vi "RGBC_init.vi"(11 "Channel Name":tag="B/I2C") -> (0 "error out":errorcluster, 3 "I2C Ref Out":T1={"myRIO Reference"={"myRIO Model"=enum."Unknown", "myRIO Hardware Reference"={"Generic FPGA Reference"=refnum, "Allow multiple opens"=FALSE}}, "I2C Channels Enum"=enum."Not Connected", "I2C Configuration"={"I2C Transfer Rate"=enum."Fast mode (400 kbps)"}})   [LabVIEW 2017]
uses:
  <vilib>/myRIO/Instrument Drivers/Onboard IO/I2C/typedefs/I2C Reference.ctl
  <vilib>/myRIO/Common/Instrument Driver Framework/Utilities/typedefs/myRIO Generic Hardware Reference.ctl
  <vilib>/myRIO/Common/Instrument Driver Framework/Utilities/typedefs/Hardware Version Enum.ctl
  <vilib>/myRIO/Common/Instrument Driver Framework/Utilities/typedefs/myRIO v1.0 Reference.ctl
  <vilib>/myRIO/Common/Instrument Driver Framework/Utilities/typedefs/Generic FPGA Reference.ctl
  <vilib>/myRIO/Common/Instrument Driver Framework/myRIO v1.0/I2C/typedefs/I2C Channels Enum.ctl
  <vilib>/myRIO/Instrument Drivers/Onboard IO/I2C/typedefs/I2C Configuration.ctl
  <vilib>/myRIO/Instrument Drivers/Onboard IO/I2C/typedefs/I2C Transfer Rate.ctl
  <vilib>/myRIO/Instrument Drivers/Onboard IO/I2C/typedefs/I2C User Configuration.ctl
  <vilib>/Utility/error.llb/Error Cluster From Error Code.vi
  <vilib>/myRIO/Common/Instrument Driver Framework/myRIO v1.0/I2C/vis/myRIO v1.0 Configure I2C.vi
  <vilib>/myRIO/Common/Instrument Driver Framework/myRIO v1.0/I2C/vis/myRIO v1.0 Write I2C.vi
  <vilib>/myRIO/Common/Instrument Driver Framework/myRIO v1.0/I2C/vis/myRIO v1.0 Read I2C.vi
  <vilib>/myRIO/Instrument Drivers/Onboard IO/I2C/I2C.lvlib
panel:
  in  "error in (no error)":errorcluster
  # "2981 EB8F 0180 0180 83"
  # "Set gain"
  # "Gain"
  # "Set enable"
  # "Enable"
  # "Set enable"
  # "Enable/timer on"
  # "Set integration time"
  # "Integration Time"
  # "Check for sensor"
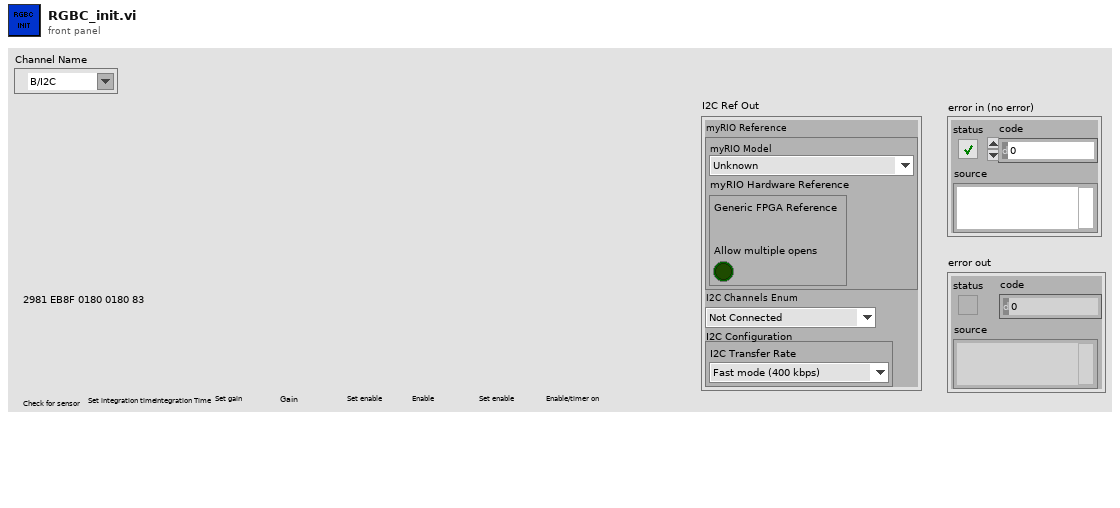
[diagram p1: front panel]
types:
  T1 = typedef "I2C.lvlib/I2C Reference.ctl" = cluster{"myRIO Reference":T2, "I2C Channels Enum":T6, "I2C Configuration":T7}
  T2 = typedef "myRIO Generic Hardware Reference.ctl" = cluster{"myRIO Model":T3, "myRIO Hardware Reference":T4}
  T3 = typedef "Hardware Version Enum.ctl" = enum16{"Unknown", "myRIO-1900", "myRIO-1950", "roboRIO", "NI ELVIS RIO CM"}
  T4 = typedef "myRIO v1.0 Reference.ctl" = cluster{"Generic FPGA Reference":T5, "Allow multiple opens":bool}
  T5 = typedef "Generic FPGA Reference.ctl" = refnum<k20>
  T6 = typedef "I2C Channels Enum.ctl" = enum16{"Not Connected", "A/I2C", "B/I2C", "I2C/I2C"}
  T7 = typedef "I2C.lvlib/I2C Configuration.ctl" = cluster{"I2C Transfer Rate":T8}
  T8 = typedef "I2C.lvlib/I2C Transfer Rate.ctl" = enum16{"Standard mode (100 kbps)", "Fast mode (400 kbps)"}
  T9 = typedef "I2C.lvlib/I2C User Configuration.ctl" = cluster{"I2C Transfer Rate":T8}
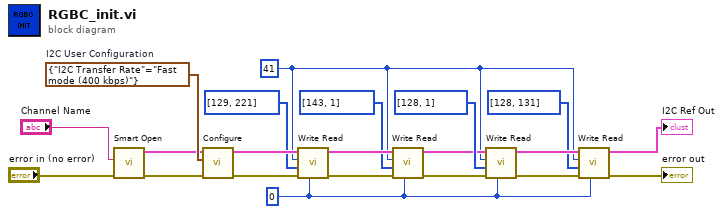
[diagram p0: block diagram]
diagram:
  w1 = u32 0 ("Byte Count")
  w4 = u8 41 ("Slave Address (7-bit)")
  w20 = T9 {"I2C Transfer Rate"=enum."Fast mode (400 kbps)"}  # I2C User Configuration
  n1 = call <vilib>:"Smart Open.vi"("error in (no error)"="error in (no error)", "Channel Name"="Channel Name") -> ("error out"=w17:errorcluster, "I2C Ref Out"=w18:T1)  [unwired: 8 in]
  n2 = call <vilib>:"Configure.vi"("error in (no error)"=w17, "I2C User Configuration"=w20, "I2C Ref In"=w18) -> ("error out"=w15:errorcluster, "I2C Ref Out"=w16:T1)  [unwired: 7 in]
  n3 = call <vilib>:"Write Read.vi"("Byte Count"=w1, "error in (no error)"=w15, "Bytes to Write"=u8[] [129, 221], "Slave Address (7-bit)"=w4, "I2C Ref In"=w16) -> ("error out"=w12:errorcluster, "I2C Ref Out"=w13:T1)  [unwired: 3 in, 1 out]
  n4 = call <vilib>:"Write Read.vi"("Byte Count"=w1, "error in (no error)"=w12, "Bytes to Write"=u8[] [143, 1], "Slave Address (7-bit)"=w4, "I2C Ref In"=w13) -> ("error out"=w8:errorcluster, "I2C Ref Out"=w9:T1)  [unwired: 3 in, 1 out]
  n5 = call <vilib>:"Write Read.vi"("Byte Count"=w1, "error in (no error)"=w8, "Bytes to Write"=u8[] [128, 1], "Slave Address (7-bit)"=w4, "I2C Ref In"=w9) -> ("error out"=w6:errorcluster, "I2C Ref Out"=w7:T1)  [unwired: 3 in, 1 out]
  n6 = call <vilib>:"Write Read.vi"("Byte Count"=w1, "error in (no error)"=w6, "Bytes to Write"=u8[] [128, 131], "Slave Address (7-bit)"=w4, "I2C Ref In"=w7) -> ("error out"=→"error out":errorcluster, "I2C Ref Out"=→"I2C Ref Out":T1)  [unwired: 3 in, 1 out]
